vi "FGV_GuideTree.vi"(7 "Action":T1, 8 "error in":errorcluster caption="错误输入（无错误）", 10 "Tag":string, 11 "Tree*":refnum<vi>) -> (0 "error out":errorcluster caption="错误输出", 2 "UIname":string, 3 "Tree* out":refnum<vi>)   [LabVIEW 2017]
uses:
  FGV_GuideTree.ctl
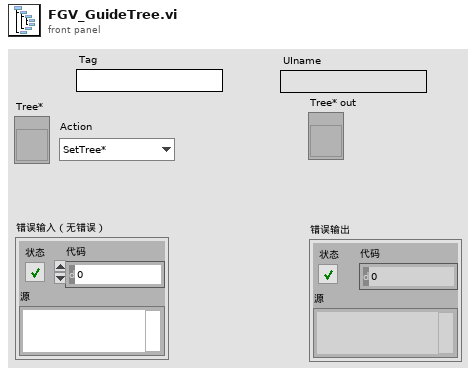
[diagram p1: front panel]
types:
  T1 = typedef "FGV_GuideTree.ctl" = enum16{"SetTree*", "GetTree*", "InitlizeTree", "Get Item infor"}
  T2 = cluster{"Left Cell String":string, "Child Text":string[], "Child Tag":string, "Item Indent":i32, "Child Only?":bool, "Glyph Index":i32}
  T3 = cluster{"Image":path, "Modules":path, "System.ini":path}
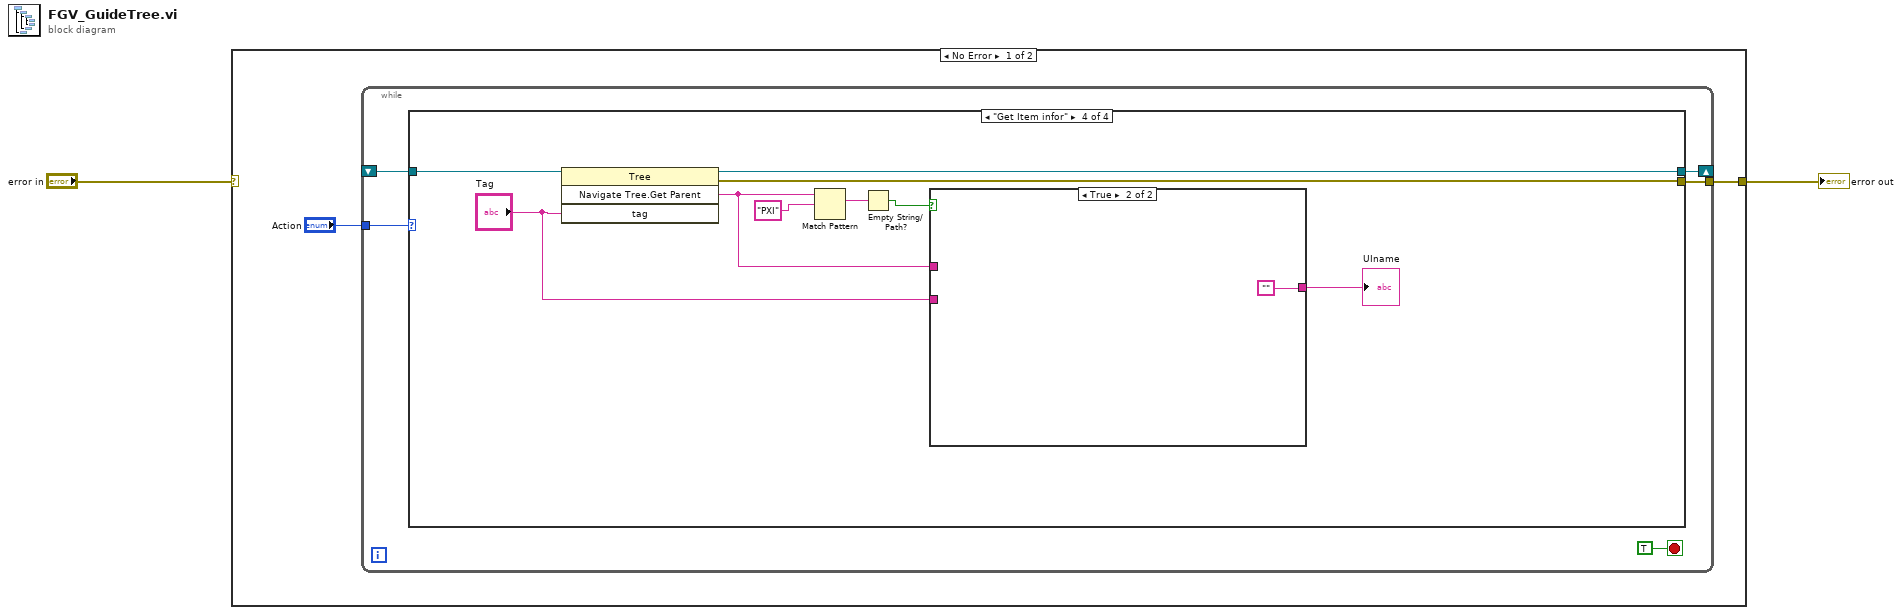
[diagram p0: block diagram]
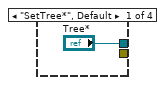
[diagram p2: hidden frame]
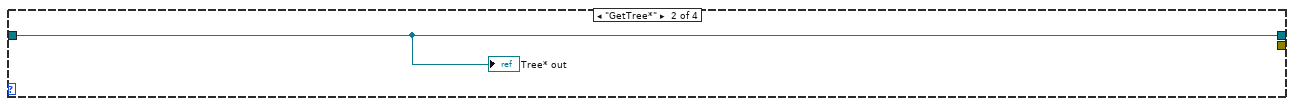
[diagram p3: hidden frame]
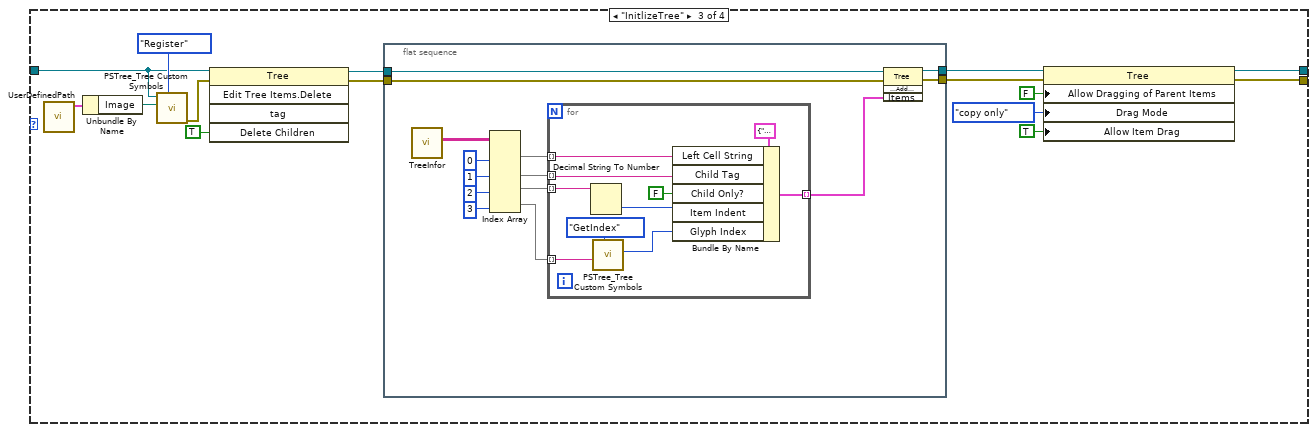
[diagram p4: hidden frame]
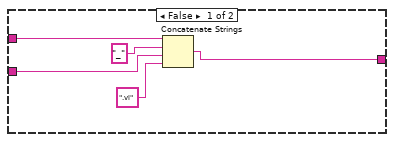
[diagram p5: hidden frame]
diagram:
  n1 = case shown="No Error" "error in" {
    selector: "error in" -> [_ w66]
    tunnel: [w3 w66] -> w2
    frame No Error {
      n2 = while {
        tunnel: "Action" -> [w8]
        shift-right: [w6] -> _
        shift-left: _ -> [w7]
        tunnel: [w5] -> w3
        stop <- TRUE stop-if-true
        n3 = case shown="\"Get Item infor\"" w8 {
          tunnel: w7 -> [_ w11 w21 w59]
          tunnel: ["Tree*" w11 w14 w58] -> w6
          tunnel: [_ _ w12 w52] -> w5
          frame "SetTree*", Default {
          }
          frame "GetTree*" {
            "Tree* out" <- w11
          }
          frame "InitlizeTree" {
            n4 = call "UserDefinedPath.vi"() -> ("ProDefPath"=w20:T3)  [unwired: 11 in]
            n5 = Unbundle By Name(w20) -> ("Image"=w19:path)
            n6 = call "PSTree_Tree Custom Symbols.vi"("Operation"=enum16{"Register", "GetIndex"}."Register", "Files"=w19, "tree refnum"=w21) -> ("error out"=w25:errorcluster)  [unwired: 7 in, 1 out]
            n7 = invoke class="Tree" method="Edit Tree Items.Delete"(reference=w21, error in=w25, "Delete Children"=TRUE ("删除子项？")) -> (reference out=w23:refnum<vi>, error out=w24:errorcluster)  [unwired: 2 in, 3 out]
            n8 = flat-sequence {
              tunnel: w24 -> [w40]
              tunnel: w23 -> [w39]
              tunnel: [w29] -> w15
              tunnel: [w28] -> w13
              frame #0 {
                n9 = call "TreeInfor.vi"() -> ("Array"=w27:string[][])  [unwired: 11 in]
                n10 = Index Array(array=w27, index (col) #1=0 ("禁用的索引 (列)"), index (col) #2=1 ("索引 (列)"), index (col) #3=2 ("索引 (列)"), index (col) #4=3 ("索引 (列)")) -> (element #1=w37:string[], element #2=w33:string[], element #3=w30:string[], element #4=w31:string[])  [unwired: 4 in]
                n11 = for {
                  tunnel: [w49] -> w35 mode=indexing
                  tunnel: w37 -> [w46] mode=indexing
                  tunnel: w31 -> [w45] mode=indexing
                  tunnel: w33 -> [w43] mode=indexing
                  tunnel: w30 -> [w42] mode=indexing
                  n12 = Decimal String To Number(string=w42) -> (number=w44:i32)  [unwired: 2 in, 1 out]
                  n13 = call "PSTree_Tree Custom Symbols.vi"("Operation"=enum16{"Register", "GetIndex"}."GetIndex", "PicName"=w45) -> ("PicIndex"=w47:i32)  [unwired: 8 in, 1 out]
                  n14 = Bundle By Name(cluster=T2 {"Left Cell String"="", "Child Text"=[], "Child Tag"="", "Item Indent"=0, "Child Only?"=FALSE, "Glyph Index"=0} ("Item"), "Left Cell String"=w46, "Child Tag"=w43, "Child Only?"=FALSE, "Item Indent"=w44, "Glyph Index"=w47) -> (w49:T2)
                }
                n15 = invoke class="Tree" method="Edit Tree Items.Add Multiple Items to End"(reference=w39, error in=w40, "Items"=w35) -> (reference out=w29:refnum<vi>, error out=w28:errorcluster)  [unwired: 1 in, 2 out]
              }
            }
            n16 = property class="Tree"(reference=w15, error in=w13, "Allow Dragging of Parent Items"=FALSE ("拖曳/放置:允许拖曳父项"), "Drag Mode"=enum32{"copy or move", "copy only", "move only"}."copy only" ("拖曳/放置:拖曳模式"), "Allow Item Drag"=TRUE ("拖曳/放置:允许拖曳")) -> (reference out=w14:refnum<vi>, error out=w12:errorcluster)
          }
          frame "Get Item infor" {
            n17 = invoke class="Tree" method="Navigate Tree.Get Parent"(reference=w59, "tag"="Tag") -> (reference out=w58:refnum<vi>, error out=w52:errorcluster, "Navigate Tree:Get Parent"=w54:string)  [unwired: 2 in, 1 out]
            n18 = Match Pattern(string=w54, regular expression="PXI") -> (match substring=w56:string)  [unwired: 1 in, 3 out]
            n19 = Empty String/Path?(string/path=w56) -> (empty?=w55:bool)
            n20 = case shown="True" w55 {
              tunnel: w54 -> [w64 _]
              tunnel: "Tag" -> [w62 _]
              tunnel: [w60 ""] -> w51
              frame False {
                n21 = Concatenate Strings(w64, "_", w62, ".vi") -> (w60:string)
              }
              frame True {
              }
            }
            "UIname" <- w51
          }
        }
      }
    }
    frame Error {
    }
  }
  "error out" <- w2
